vi "Configure Clock Recovery.vi"   [LabVIEW 2015, in "Agilent 2000 3000 X-Series.lvlib"]
doc: "Clock Recovery Polymorphic VI"
uses:
  <instrlib>/Agilent 2000 3000 X-Series/Agilent 2000 3000 X-Series.lvlib
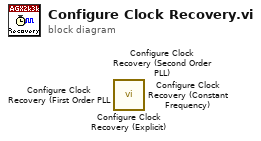
[diagram p0: block diagram]
diagram:
  n1 = call <instrlib>:"Configure Clock Recovery (Explicit).vi"() -> ()  [unwired: 10 in, 2 out]
  n2 = call <instrlib>:"Configure Clock Recovery (Second Order PLL).vi"() -> ()  [unwired: 10 in, 2 out]
  n3 = call <instrlib>:"Configure Clock Recovery (First Order PLL.vi"() -> ()  [unwired: 10 in, 2 out]
  n4 = call <instrlib>:"Configure Clock Recovery (Constant Frequency).vi"() -> ()  [unwired: 10 in, 2 out]
